vi "ABR3-Is Stimulus Stereo Wav File.vi"(0 "Stimulus":T2={"Ear"=enum."Left", "Waveform"=enum."TONE PIP", "Frequency (kHz)"="", "Rep rate (/sec)"=30.0, "Alternate Polarity"=FALSE, "WavFiles"="", "Level (dB SPL)"=30.0, "WavFolder"=path "", "Chirp"={"Type"=enum."AN latency-corrected", "Duration (ms)"=0.0, "Fmin (kHz)"=0.0, "Fmax (kHz)"=0.0, "precompensate"=FALSE}, "Noise"={"Seed"=0, "InvFilt"=FALSE, "AWeight"=FALSE, "afile"=path "", "Filter"={"Type"=enum."Lowpass", "CF (kHz)"=0.0, "BW (kHz)"=0.0, "Cascade"=FALSE, "Quadrature"=FALSE, "Scale Factor"=0.0, "Stages"=[], "Class"=enum."Elliptic", "Order"=0, "BWUnits"=enum."Linear"}}}) -> (1 "Is Stereo Wav File":bool, 2 "Channel To Add":T1)   [LabVIEW 2020]
uses:
  TypeDefs/ABR3-Stimulus.ctl
  epl-vi-lib/Utility VIs/Type Defs/Left-Right ring.ctl
  TypeDefs/ABR-Waveform Enum.ctl
  epl-vi-lib/Signal Synthesis VIs/Controls/Advanced Filter XCtl/Advanced Filter XCtl.xctl
  epl-vi-lib/Utility VIs/Type Defs/Speaker ring.ctl
  <vilib>/sound2/lvsound2.llb/Sound File Info (path).vi
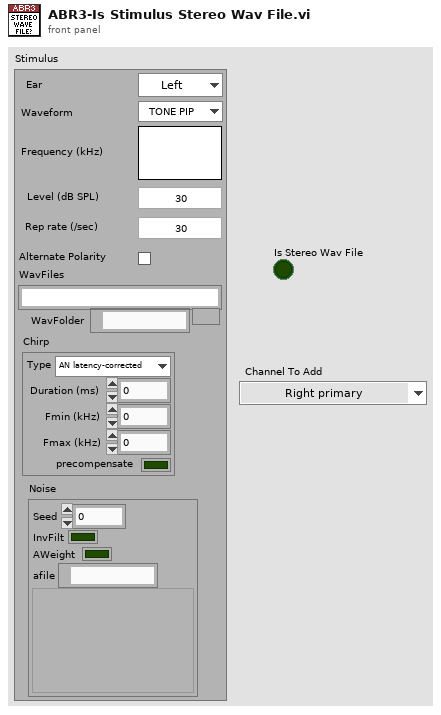
[diagram p1: front panel]
types:
  T1 = typedef "Speaker ring.ctl" = enum16{"Right primary", "Right secondary", "Left primary", "Left secondary"}
  T2 = typedef "ABR3-Stimulus.ctl" = cluster{"Ear":T3, "Waveform":T4, "Frequency (kHz)":string, "Rep rate (/sec)":dbl, "Alternate Polarity":bool, "WavFiles":string, "Level (dB SPL)":dbl, "WavFolder":path, "Chirp":cluster{"Type":enum16{"AN latency-corrected", "Arbitrary"}, "Duration (ms)":dbl, "Fmin (kHz)":dbl, "Fmax (kHz)":dbl, "precompensate":bool}, "Noise":cluster{"Seed":i32, "InvFilt":bool, "AWeight":bool, "afile":path, "Filter":cluster{"Type":enum16{"Lowpass", "Highpass", "Bandpass", "Bandstop", "OFF"}, "CF (kHz)":dbl, "BW (kHz)":dbl, "Cascade":bool, "Quadrature":bool, "Scale Factor":dbl, "Stages":cluster{"IIR Filter":cluster{"filter structure":enum32{"IIR 2nd Order", "IIR 4th Order"}, "Reverse Coefficients":dbl[], "Forward Coefficients":dbl[]}, "State":dbl[]}[], "Class":enum16{"Elliptic", "Butterworth"}, "Order":i32, "BWUnits":T5}}}
  T3 = typedef "Left-Right ring.ctl" = enum16{"Right", "Left"}
  T4 = typedef "ABR-Waveform Enum.ctl" = enum16{"TONE PIP", "CLICK", "FILE", "CHIRP", "NOISE", "VERHULST"}
  T5 = typedef "Filter-Bandwidth Units.ctl" = enum16{"Linear", "Octaves", "Min-Max"}
  T6 = typedef "Sound Data Format.ctl" = cluster{"sample rate (S/s)":dbl, "number of channels":i32, "bits per sample":i32}
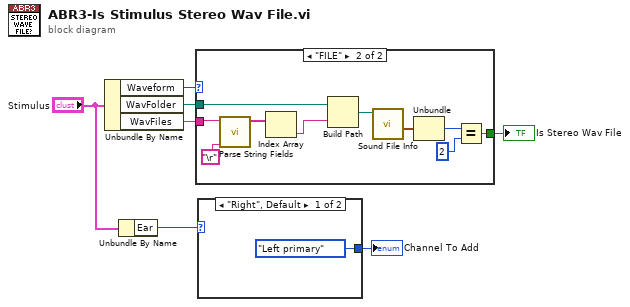
[diagram p0: block diagram]
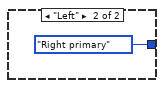
[diagram p2: hidden frame]
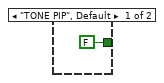
[diagram p3: hidden frame]
diagram:
  n1 = Unbundle By Name("Stimulus") -> ("Waveform"=w5:T4, "WavFolder"=w6:path, "WavFiles"=w7:string)
  n2 = Unbundle By Name("Stimulus") -> ("Ear"=w2:T3)
  n3 = case shown="\"FILE\"" w5 {
    tunnel: w7 -> [_ w17]
    tunnel: w6 -> [_ w18]
    tunnel: [FALSE w9] -> w4
    frame "TONE PIP", Default {
    }
    frame "FILE" {
      n4 = call "Parse String Fields.vi"("Separator"="\r", "String"=w17) -> ("Fields"=w15:string[])  [unwired: 8 in, 1 out]
      n5 = Index Array(array=w15) -> (element=w14:string)  [unwired: 1 in]
      n6 = Build Path(base path=w18, name or relative path=w14) -> (appended path=w12:path)
      n7 = call-poly <vilib>:"Sound File Info.vi"("path"=w12) -> ("sound format"=w13:T6)  [unwired: 7 in, 3 out]
      n8 = Unbundle(w13) -> ("number of channels"=w11:i32)  [unwired: 2 out]
      n9 = Equal?(x=w11, y=2) -> (x = y?=w9:bool)
    }
  }
  "Is Stereo Wav File" <- w4
  n10 = case shown="\"Right\", Default" w2 {
    tunnel: [Speaker_ring."Left primary" ("Speaker") Speaker_ring."Right primary" ("Speaker")] -> w1
    frame "Right", Default {
    }
    frame "Left" {
    }
  }
  "Channel To Add" <- w1
